vi "Event Actor.vi"(4 "Queue Nested":map{string, refnum<data-value>}(c390), 6 "Queue Self":map{string, refnum<data-value>}(c390), 8 "Queue Caller":map{string, refnum<data-value>}(c390), 9 "Queue of Event Self":refnum<queue>, 10 "Event Self Alias":string, 11 "Event Actor":refnum<class "Event Actor.lvclass">) -> ()   [LabVIEW 2021, in "jettl.lvlib" / "jettl Event Actor.lvlib" / "jettl Event Actor.lvclass"]
uses:
  jettl Event Actor.lvclass
  Actor/Event Actor/Event Actor.lvclass
  Actor/Msg/Msg.lvclass
  Actor/Msgs/Setup/Setup Msg/Setup Msg.lvclass
  C:/git/jettl/src/Actor/Msg/Msg.lvclass
  C:/git/jettl/src/Actor/Event Actor/Event Actor.lvclass
  Actor/Msgs/Event Last Ack/Event Last Ack Msg/Event Last Ack Msg.lvclass
  jettl.lvlib
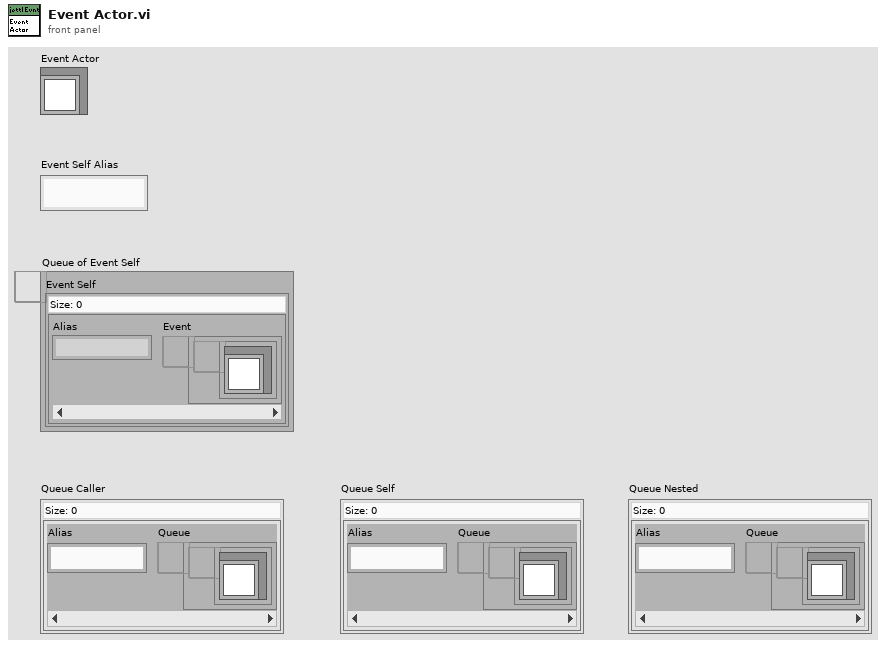
[diagram p1: front panel]
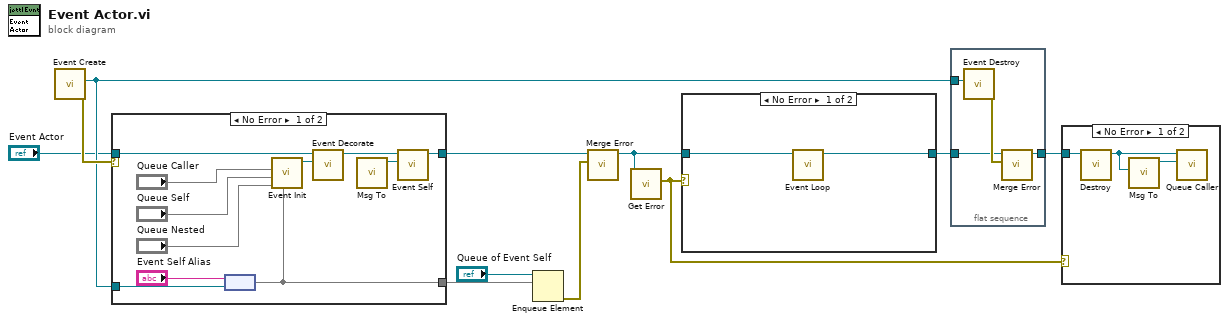
[diagram p0: block diagram]
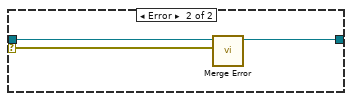
[diagram p3: hidden frame]
diagram:
  n1 = call "Event Create.vi"() -> ("error out"=w4:errorcluster, "Event"=w3:refnum<data-value>)  [unwired: 10 in]
  n2 = case shown="No Error" w4 {
    selector: w4 -> [_ w24]
    tunnel: [w13 w25] -> w8
    tunnel: "Event Actor" -> [w21 w23]
    tunnel: w3 -> [w22 _]
    tunnel: [w19 _] -> w7
    frame No Error {
      n3 = node("Event Self Alias", w22) -> (w19:map{string, refnum<data-value>})
      n4 = call "Event Init.vi"("Event Self"=w19, "Queue Nested"="Queue Nested", "Queue Self"="Queue Self", "Queue Caller"="Queue Caller") -> ("jettl Event Actor out"=w20:refnum<class "jettl Event Actor.lvclass">)  [unwired: 7 in]
      n5 = call-dynamic "Event Decorate.vi"("Event Actor"=w20, "Event Actor in"=w21) -> ("Event Actor out"=w14:refnum<class "Event Actor.lvclass">)  [unwired: 9 in]
      n6 = call "Msg To.vi"() -> ("Setup Msg out"=w12:refnum<class "Setup Msg.lvclass">)  [unwired: 11 in]
      n7 = call-dynamic "Event Self.vi"("Msg"=w12, "Event Actor in"=w14) -> ("Event Actor out"=w13:refnum<class "Event Actor.lvclass">)  [unwired: 9 in]
    }
    frame Error {
      n8 = call-dynamic "Merge Error.vi"("Error"=w24, "Set Error in"=w23) -> ("Set Error out"=w25:refnum<class "Event Actor.lvclass">)  [unwired: 9 in]
    }
  }
  n9 = Enqueue Element(queue="Queue of Event Self", element=w7) -> (error out=w9:errorcluster)  [unwired: 2 in, 2 out]
  n10 = call-dynamic "Merge Error.vi"("Error"=w9, "Set Error in"=w8) -> ("Set Error out"=w10:refnum<class "Event Actor.lvclass">)  [unwired: 9 in]
  n11 = call-dynamic "Get Error.vi"("Actor in"=w10) -> ("Error"=w6:errorcluster)  [unwired: 10 in]
  n12 = case shown="No Error" w6 {
    tunnel: w10 -> [w27 w28]
    tunnel: [w26 w28] -> w5
    frame No Error {
      n13 = call-dynamic "Event Loop.vi"("Event Actor in"=w27) -> ("Event Actor out"=w26:refnum<class "Event Actor.lvclass">)  [unwired: 10 in]
    }
    frame Error {
    }
  }
  n14 = flat-sequence {
    tunnel: w3 -> [w31]
    tunnel: [w32] -> w11
    tunnel: w5 -> [w29]
    frame #0 {
      n15 = call "Event Destroy.vi"("Event"=w31) -> ("error out"=w30:errorcluster)  [unwired: 10 in]
      n16 = call-dynamic "Merge Error.vi"("Error"=w30, "Set Error in"=w29) -> ("Set Error out"=w32:refnum<class "Event Actor.lvclass">)  [unwired: 9 in]
    }
  }
  n17 = case shown="No Error" w6 {
    tunnel: w11 -> [w35 _]
    frame No Error {
      n18 = call-dynamic "Destroy.vi"("Actor in"=w35) -> ("Actor out"=w33:refnum<class "Event Actor.lvclass">)  [unwired: 10 in]
      n19 = call "Msg To.vi"("Event Actor"=w33) -> ("Event Last Ack Msg out"=w34:refnum<class "Event Last Ack Msg.lvclass">)  [unwired: 10 in]
      n20 = call-dynamic "Queue Caller.vi"("Msg"=w34, "Actor in"=w33) -> ()  [unwired: 9 in, 1 out]
    }
    frame Error {
    }
  }
